vi "Parity to Stop Bits.vi"(11 "parity":T1 items=["None", "Odd", "Even", "Mark", "Space"]) -> (3 "Stop Bits":u32)   [LabVIEW 2015, in "Modbus Master System Explorer.lvlib"]
uses:
  Modbus Master System Explorer.lvlib
  Shared/Controls/Parity.ctl
  Shared/Modbus Master Shared.lvlib
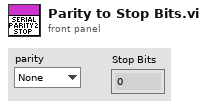
[diagram p1: front panel]
types:
  T1 = typedef "Modbus Master Shared.lvlib/Parity.ctl" = u16
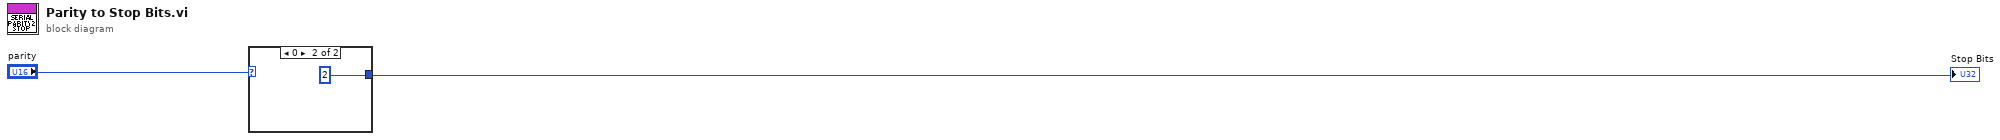
[diagram p0: block diagram]
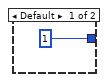
[diagram p2: hidden frame]
diagram:
  n1 = case shown="0" "parity" {
    tunnel: [u32 1 ("Data Bits") u32 2 ("Data Bits")] -> w2
    frame Default {
    }
    frame 0 {
    }
  }
  "Stop Bits" <- w2
